vi "MainStateMachine.vi"(8 "error constant":errorcluster, 11 "FPGA VI Reference In":refnum<k20>) -> (0 "error constant 2":errorcluster, 3 "FPGA VI Reference Out":refnum<k20>)   [LabVIEW 2018]
uses:
  <vilib>/platform/TimedLoop/XDataNode/XDataNode.xnode
  <vilib>/Platform/TimedLoop/XDataNode/nitl_modes.ctl
  <vilib>/Platform/TimedLoop/XDataNode/XDNodeRunTimeDep.lvlib
  <vilib>/Platform/TimedLoop/XDataNode/wakeup.ctl
  <vilib>/Platform/TimedLoop/XDataNode/timing_clust.ctl
  Type_Def/Type_Def ControlState.ctl
  <vilib>/Platform/TimedLoop/XDataNode/loadnilvce.vi
  Type_Def/Type_Def Actuator Controls.ctl
  Type_Def/Type_Def AllSensorData.ctl
  2019_CompetitionCode-master/2019_CompetitionCode-master/Master/DAQ/TypeDef_cRIOData.ctl
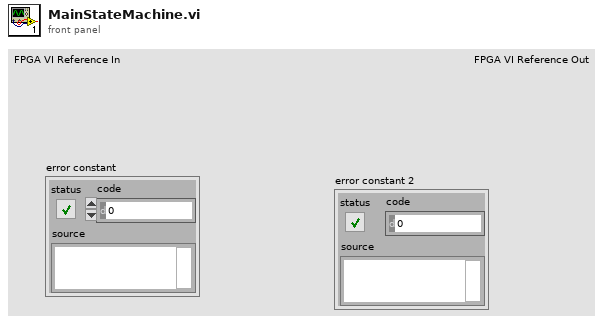
[diagram p1: front panel]
types:
  T1 = typedef "Type_Def Actuator Controls.ctl" = cluster{"Reverse ":bool, "Forward":bool, "Low Side":bool, "Precharge":bool, "High Side":bool, "Digital Out 5":bool, "Digital Out 6":bool, "Digital Out 7 ":bool, "24 Power":bool, "Tank Valve ":bool, "Brake Valve":bool, "Pump":bool, "Digital Out 1 ":bool, "Digital Out 2":bool, "Digital Out 3":bool, "Digital Out 4 ":bool}
  T2 = typedef "Type_Def ControlState.ctl" = enum16{"Blank", "Systems Check", "Idle", "Ready", "Pushing", "CrawlingPrecharge", "Braking", "Fault", "Boot Up", "Unpowered", "Crawling", "Shutdown", "Service Push", "Service Wait", "Vent", "Precharge", "Cooldown"}
  T3 = typedef "Type_Def AllSensorData.ctl" = cluster{"cRIO Data":T4}
  T4 = typedef "TypeDef_cRIOData.ctl" = cluster{"Time (ms)":dbl, "24V Battery (V)":dbl, "LowV Current (A)":dbl, "Fiducial Sensor (V)":dbl, "PV Pressure (psig)":dbl, "Flow Sensor (V)":dbl, "Temp Fairing (F)":dbl, "Temp Reservoir (F)":dbl, "HallEffect Right (in)":dbl, "HallEffect Left (in)":dbl, "PT Tank (psig)":dbl, "PT Clamp Right (psig)":dbl, "PT Clamp Left (psig)":dbl, "PT Brake (psig)":dbl, "PT Cooling (psig)":dbl, "Displacement (ft)":dbl, "Velocity (ft/s)":dbl}
  T5 = typedef "Type_Def ClusterSensor.ctl" = cluster{"Sensor Data":dbl, "Max":dbl, "Min":dbl, "Previous Data":dbl, "#same":dbl}
  T6 = typedef "XDNodeRunTimeDep.lvlib/timing_clust.ctl" = cluster{"Expected End [f-1]":u64, "Actual End [f-1]":u64, "Finished Late? [f-1]":bool, "Expected End [i-1]":u64, "Actual End [i-1]":u64, "Finished Late? [i-1]":bool, "Expected Start [i]":u64, "Actual Start [i]":u64, "Expected Start [f]":u64, "Actual Start [f]":u64, "Source Name":string, "Structure Name":string, "Period":i64, "Deadline":i64, "Offset":i64, "Start":i64, "Priority":i32, "Timeout":i32, "Mode":T7, "Wakeup Reason":T8, "Error":errorcluster, "Source Type":string, "Secondary Source Type":string, "Global End Time":u64, "Global Start Time":u64, "Frame Duration":u64, "Iteration Duration":u64, "Assigned CPU":i32, "I/O Scan Engine Mode":u32}
  T7 = typedef "XDNodeRunTimeDep.lvlib/nitl_modes.ctl" = enum32{"No Change", "Process missed periods, maintain original phase", "Discard missed periods, maintain original phase", "Process missed periods, ignore original phase", "Discard missed periods, ignore original phase"}
  T8 = typedef "XDNodeRunTimeDep.lvlib/wakeup.ctl" = enum32{"Normal", "Aborted", "Asynchronous wakeup", "Timing source error", "Timed loop error", "Timeout"}
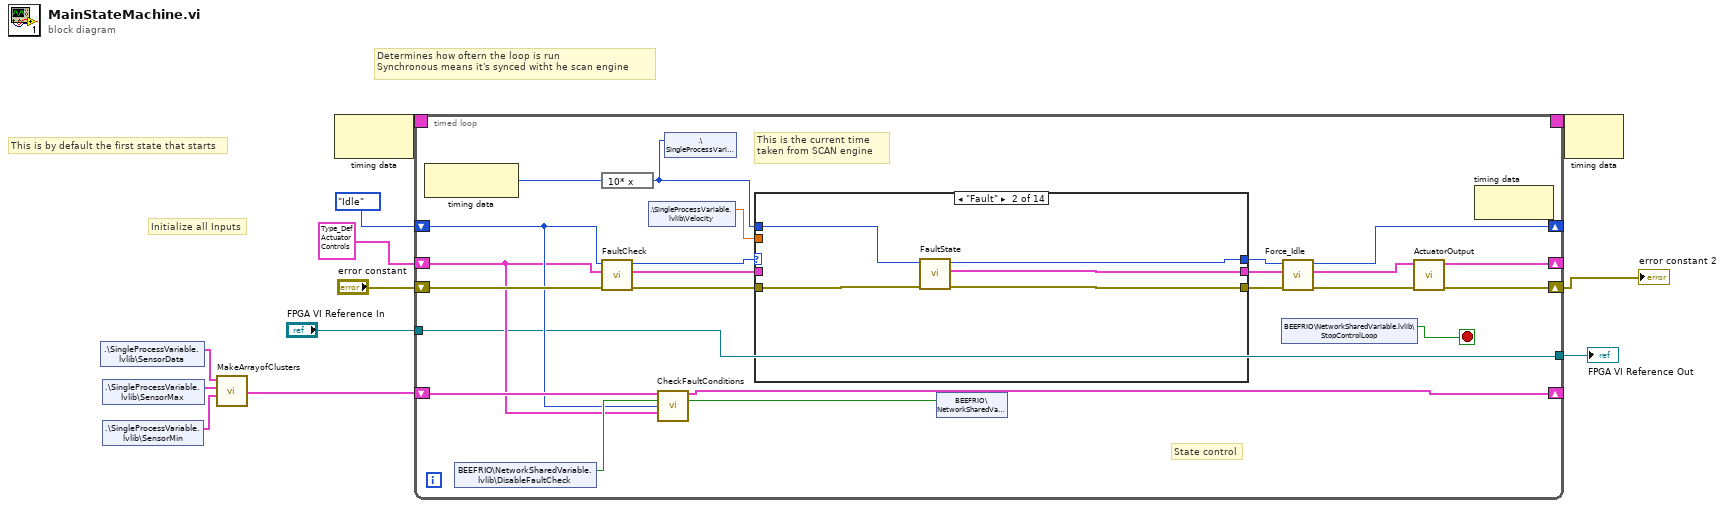
[diagram p0: block diagram]
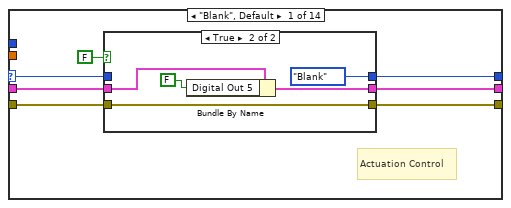
[diagram p2: hidden frame]
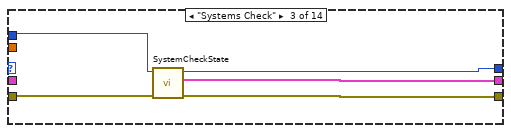
[diagram p4: hidden frame]
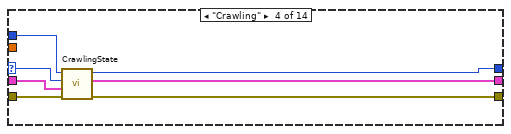
[diagram p5: hidden frame]
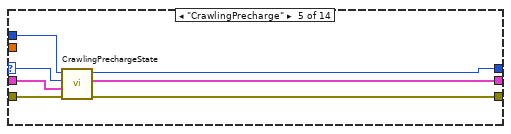
[diagram p6: hidden frame]
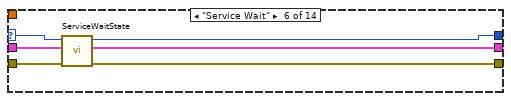
[diagram p7: hidden frame]
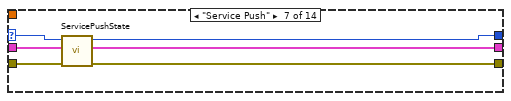
[diagram p8: hidden frame]
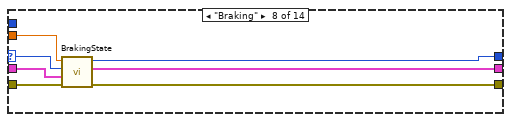
[diagram p9: hidden frame]
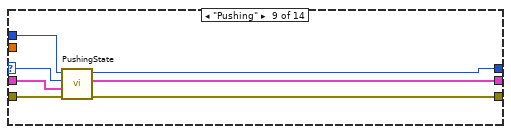
[diagram p10: hidden frame]
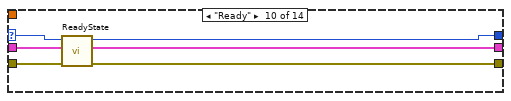
[diagram p11: hidden frame]
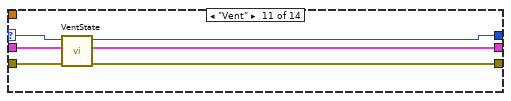
[diagram p12: hidden frame]
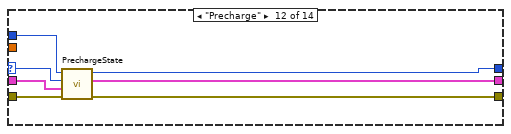
[diagram p13: hidden frame]
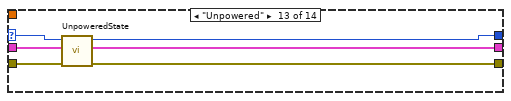
[diagram p14: hidden frame]
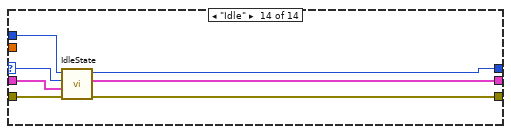
[diagram p15: hidden frame]
diagram:
  # "Determines how oftern the loop is run \nSynchronous means it's synced witht he scan engine"
  # "Initialize all Inputs"
  # "This is by default the first state that starts"
  n1 = shared-variable ".\\SingleProcessVariable.lvlib\\SensorData"() -> (w7:T3)  [unwired: 1 in, 1 out]
  n2 = shared-variable ".\\SingleProcessVariable.lvlib\\SensorMax"() -> (w6:T3)  [unwired: 1 in, 1 out]
  n3 = shared-variable ".\\SingleProcessVariable.lvlib\\SensorMin"() -> (w5:T3)  [unwired: 1 in, 1 out]
  n4 = call "MakeArrayofClusters.vi"(9:w5, 10:w6, 11:w7) -> ("Array"=w4:cluster{"SensorCluster":T5}[])  [unwired: 8 in]
  n5 = node-c288 ("Input Node")() -> (w12:T6)  [unwired: 1 in]
  n6 = timed-loop "Timed Loop" {
    timing: w12 -> [_]
    timing-out: [_] -> w11
    shift-right: [w17] -> _
    shift-left: Type_Def_ControlState."Idle" -> [w20]
    shift-right: [w29] -> _
    shift-left: T1 {"Reverse "=FALSE, "Forward"=FALSE, "Low Side"=FALSE, "Precharge"=FALSE, "High Side"=FALSE, "Digital Out 5"=FALSE, "Digital Out 6"=FALSE, "Digital Out 7 "=FALSE, "24 Power"=FALSE, "Tank Valve "=FALSE, "Brake Valve"=FALSE, "Pump"=FALSE, "Digital Out 1 "=FALSE, "Digital Out 2"=FALSE, "Digital Out 3"=FALSE, "Digital Out 4 "=FALSE} -> [w18]
    shift-right: [w28] -> w1
    shift-left: "error constant" -> [w35]
    shift-right: [w23] -> _
    shift-left: w4 -> [w22]
    tunnel: [w13] -> w3
    tunnel: "FPGA VI Reference In" -> [w13]
    stop <- w14 stop-if-true
    # "State control"
    # "This is the current time \ntaken from SCAN engine"
    n7 = node-c288() -> (w31:i64)  [unwired: 1 in]
    n8 = shared-variable "BEEFRIO\\NetworkSharedVariable.lvlib\\DisableFaultCheck"() -> (w21:bool)  [unwired: 1 in, 1 out]
    n9 = expression code="10* x"(w31) -> (w30:i64)
    n10 = call "FaultCheck.vi"("error in (no error)"=w35, "Cluster in"=w18, "Enum in"=w20) -> ("error out"=w24:errorcluster, "Cluster out"=w25:T1, "Enum out"=w26:T2)  [unwired: 6 in]
    n11 = shared-variable ".\\SingleProcessVariable.lvlib\\Velocity"() -> (w27:dbl)  [unwired: 1 in, 1 out]
    n12 = call "CheckFaultConditions.vi"("Array 2"=w22, "DisableFaultCheck"=w21, "ControlState"=w20, "Cluster"=w18) -> ("Array out"=w23:cluster{"SensorCluster":T5}[], "Fault?"=w19:bool)  [unwired: 10 in]
    n13 = shared-variable ".\\SingleProcessVariable.lvlib\\Time"(w30) -> ()  [unwired: 1 in, 1 out]
    n14 = case shown="\"Fault\"" w26 {
      selector: w26 -> [w42 _ _ w67 w74 w80 w86 w93 w100 w106 w112 w119 w125 w132]
      tunnel: [w41 w53 w58 w66 w73 w79 w85 w92 w99 w105 w111 w118 w124 w131] -> w32
      tunnel: [w39 w51 w56 w64 w71 w77 w83 w90 w97 w103 w109 w116 w122 w129] -> w34
      tunnel: w25 -> [w40 _ _ w65 w72 w78 w84 w91 w98 w104 w110 w117 w123 w130]
      tunnel: [w38 w52 w57 w63 w70 w76 w82 w89 w96 w102 w108 w115 w121 w128] -> w33
      tunnel: w24 -> [w37 w55 w59 w62 w69 w75 w81 w88 w95 w101 w107 w114 w120 w127]
      tunnel: w30 -> [_ w54 w60 w61 w68 _ _ _ w94 _ _ w113 _ w126]
      tunnel: w27 -> [_ _ _ _ _ _ _ w87 _ _ _ _ _ _]
      frame "Blank", Default {
        # "Actuation Control"
        n15 = case shown="True" FALSE {
          tunnel: w42 -> [w45 _]
          tunnel: [w45 Type_Def_ControlState."Blank"] -> w41
          tunnel: w40 -> [w44 w49]
          tunnel: [w44 w47] -> w39
          tunnel: [w43 w46] -> w38
          tunnel: w37 -> [w43 w46]
          frame False {
          }
          frame True {
            n16 = Bundle By Name(cluster=w49, "Digital Out 5"=FALSE) -> (w47:T1)
          }
        }
      }
      frame "Fault" {
        n17 = call "FaultState.vi"("error in (no error)"=w55, "Actual Start [i]"=w54) -> ("error out"=w52:errorcluster, "Cluster"=w51:T1, "Numeric"=w53:i64)  [unwired: 7 in]
      }
      frame "Systems Check" {
        n18 = call "SystemCheckState.vi"("error in (no error)"=w59, "Actual Start [i]"=w60) -> ("error out"=w57:errorcluster, "Cluster"=w56:T1, "Numeric"=w58:i64)  [unwired: 7 in]
      }
      frame "Crawling" {
        n19 = call "CrawlingState.vi"("error in (no error)"=w62, "Cluster in"=w65, "Enum in"=w67, "Actual Start [i]"=w61) -> ("error out"=w63:errorcluster, "Cluster out"=w64:T1, "Enum"=w66:T2)  [unwired: 5 in]
      }
      frame "CrawlingPrecharge" {
        n20 = call "CrawlingPrechargeState.vi"("error in (no error)"=w69, "Cluster in"=w72, "Enum in"=w74, "Actual Start [i]"=w68) -> ("error out"=w70:errorcluster, "Cluster out"=w71:T1, "Enum"=w73:T2)  [unwired: 5 in]
      }
      frame "Service Wait" {
        n21 = call "ServiceWaitState.vi"("error in (no error)"=w75, "Cluster in"=w78, "Enum in"=w80) -> ("error out"=w76:errorcluster, "Cluster out"=w77:T1, "Enum"=w79:T2)  [unwired: 6 in]
      }
      frame "Service Push" {
        n22 = call "ServicePushState.vi"("error in (no error)"=w81, "Cluster in"=w84, "Enum in"=w86) -> ("error out"=w82:errorcluster, "Cluster out"=w83:T1, "Enum out"=w85:T2)  [unwired: 6 in]
      }
      frame "Braking" {
        n23 = call "BrakingState.vi"("error in (no error)"=w88, "Cluster in"=w91, "Enum in"=w93, "Double"=w87) -> ("error out"=w89:errorcluster, "Cluster"=w90:T1, "Enum"=w92:T2)  [unwired: 5 in]
      }
      frame "Pushing" {
        n24 = call "PushingState.vi"("error in (no error)"=w95, "Cluster in"=w98, "Enum in"=w100, "Actual Start [i]"=w94) -> ("error out"=w96:errorcluster, "Cluster out"=w97:T1, "Enum"=w99:T2)  [unwired: 5 in]
      }
      frame "Ready" {
        n25 = call "ReadyState.vi"("error in (no error)"=w101, "Cluster in"=w104, "Enum in"=w106) -> ("error out"=w102:errorcluster, "Cluster out"=w103:T1, "Enum"=w105:T2)  [unwired: 6 in]
      }
      frame "Vent" {
        n26 = call "VentState.vi"("error in (no error)"=w107, "Cluster in"=w110, "Enum in"=w112) -> ("error out"=w108:errorcluster, "Cluster out"=w109:T1, "Enum out"=w111:T2)  [unwired: 6 in]
      }
      frame "Precharge" {
        n27 = call "PrechargeState.vi"("error in (no error)"=w114, "Cluster in"=w117, "Enum in"=w119, "Actual Start [i]"=w113) -> ("error out"=w115:errorcluster, "Cluster out"=w116:T1, "Enum"=w118:T2)  [unwired: 5 in]
      }
      frame "Unpowered" {
        n28 = call "UnpoweredState.vi"("error in (no error)"=w120, "Cluster in"=w123, "Enum in"=w125) -> ("error out"=w121:errorcluster, "Cluster out"=w122:T1, "Enum"=w124:T2)  [unwired: 6 in]
      }
      frame "Idle" {
        n29 = call "IdleState.vi"("error in (no error)"=w127, "Cluster in"=w130, "Enum in"=w132, "Actual Start [i]"=w126) -> ("error out"=w128:errorcluster, "Cluster out"=w129:T1, "Enum"=w131:T2)  [unwired: 5 in]
      }
    }
    n30 = shared-variable "BEEFRIO\\NetworkSharedVariable.lvlib\\Fault"(w19) -> ()  [unwired: 1 in, 1 out]
    n31 = shared-variable "BEEFRIO\\NetworkSharedVariable.lvlib\\StopControlLoop"() -> (w14:bool)  [unwired: 1 in, 1 out]
    n32 = call "Force_Idle.vi"("error in (no error)"=w33, "Cluster in"=w34, "Enum in"=w32) -> ("error out"=w15:errorcluster, "Cluster out"=w16:T1, "Enum out"=w17:T2)  [unwired: 6 in]
    n33 = call "ActuatorOutput.vi"("error in (no error)"=w15, "Cluster in"=w16) -> ("error out"=w28:errorcluster, "Cluster"=w29:T1)  [unwired: 8 in]
    n34 = node-c288() -> ()  [unwired: 1 in, 1 out]
  }
  "FPGA VI Reference Out" <- w3
  "error constant 2" <- w1
  n35 = node-c288(w11) -> ()  [unwired: 1 out]
